vi "_Unlock JKISMQ.vi"(8 "Error in":errorcluster caption="Error in (no error)", 11 "JKISMQ in":T1) -> (0 "Error out":errorcluster, 3 "JKISMQ out":T1)   [LabVIEW 2014, in "JKI State Machine++.lvlib"]
uses:
  JKI State Machine++.lvlib
  _JKISMQ.ctl
  Typedef/_Cross JKISM State Data.ctl
  Typedef/_JKISM_MSG_TYPE.ctl
  Typedef/_Cross JKISM State Response.ctl
  Typedef/_JKISM_MODE.ctl
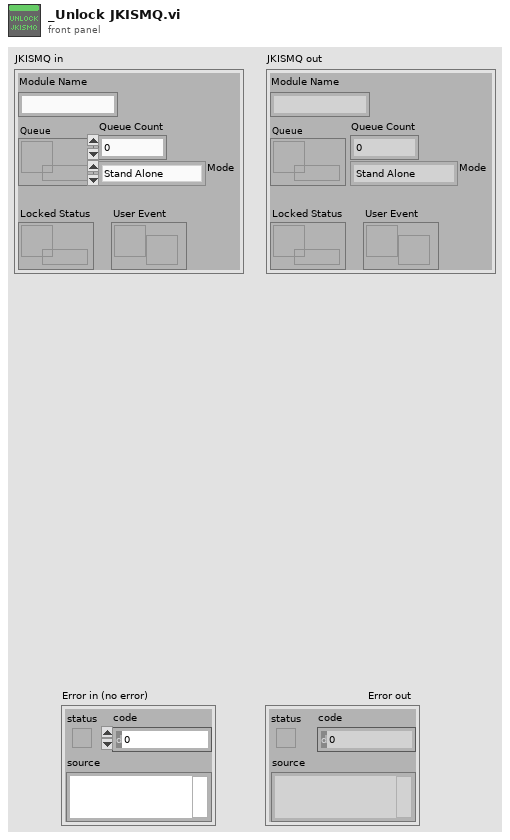
[diagram p1: front panel]
types:
  T1 = typedef "JKI State Machine++.lvlib/_JKISMQ.ctl" = cluster{"Module Name":string, "Queue":refnum<queue>, "Locked Status":refnum<data-value>, "Mode":T2, "User Event":refnum<user-event>, "Queue Count":i32}
  T2 = typedef "JKI State Machine++.lvlib/_JKISM_MODE.ctl" = enum16{"Stand Alone", "JKISM", "Action Worker"}
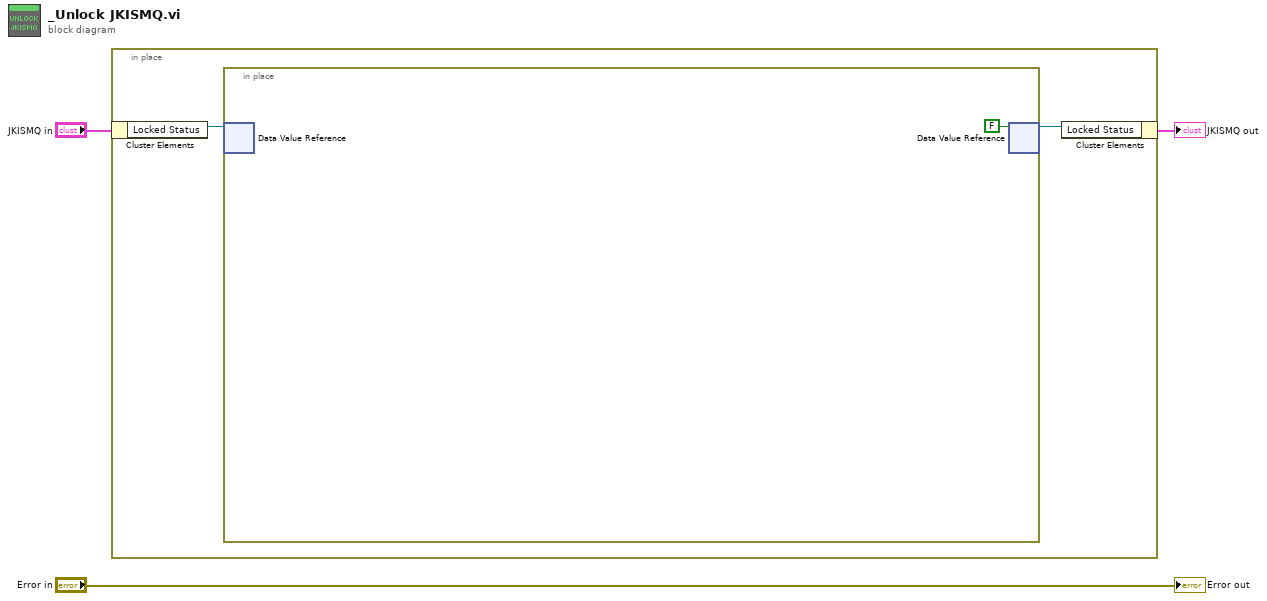
[diagram p0: block diagram]
diagram:
  n1 = in-place "In Place Element Structure" {
    n2 = in-place-cluster #1("JKISMQ in") -> ("Locked Status"=w5:refnum<data-value>)
    n3 = in-place {
      n4 = in-place-dvr #2(w5) -> ()  [unwired: 2 out]
      n5 = in-place-dvr #2(FALSE ("data value")) -> (w4:refnum<data-value>)  [unwired: 1 out]
    }
    n6 = in-place-cluster #1("Locked Status"=w4) -> (→"JKISMQ out":T1)
  }
  "Error out" <- "Error in"
